vi "Get Movie Paths.vi"(8 "error in (no error)":errorcluster, 11 "Protocol in":refnum<class "Protocol.lvclass">) -> (0 "error out":errorcluster, 2 "Paths":path[](array[path]), 3 "Protocol out":refnum<class "Protocol.lvclass">)   [LabVIEW 2023]
uses:
  Protocol.lvclass
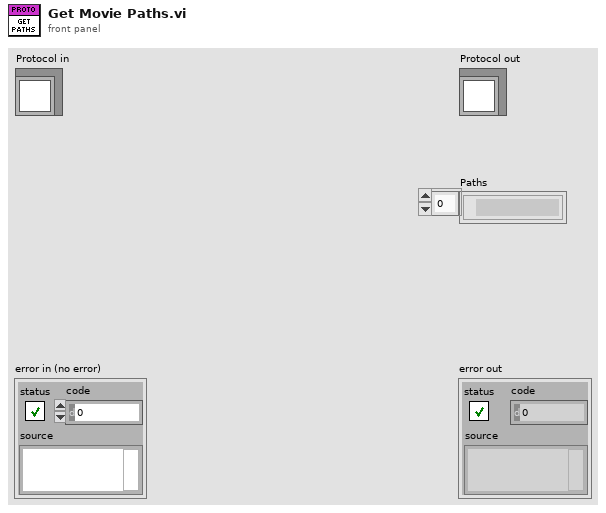
[diagram p1: front panel]
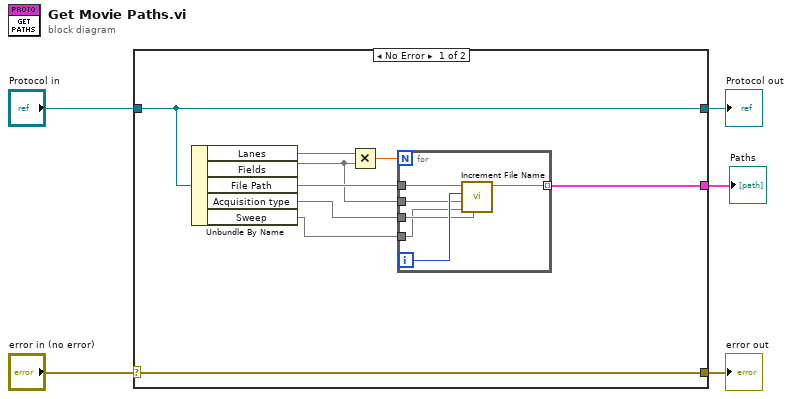
[diagram p0: block diagram]
diagram:
  n1 = case shown="No Error" "error in (no error)" {
    selector: "error in (no error)" -> [w14 w22]
    tunnel: [w14 w22] -> w4
    tunnel: [w13 w21] -> w2
    tunnel: "Protocol in" -> [w13 w21]
    tunnel: [w7 _] -> w1
    frame No Error {
      n2 = Unbundle By Name(w13) -> ("Lanes"=w11, "Fields"=w8, "File Path"=w12, "Acquisition type"=w9, "Sweep"=w6)
      n3 = Multiply(x=w11, y=w8) -> (x*y=w10:dbl)
      n4 = for {
        N: w10 -> [_]
        tunnel: w12 -> [w20]
        tunnel: w8 -> [w18]
        tunnel: w9 -> [w17]
        tunnel: [w16] -> w7 mode=indexing
        tunnel: w6 -> [w15]
        i -> [w19]
        n5 = call "Increment File Name.vi"(6:w17, 8:w15, 9:w18, "Movie Index"=w19, "Movie Series In"=w20) -> (3:w16)  [unwired: 5 in, 1 out]
      }
    }
    frame Error {
    }
  }
  "error out" <- w4
  "Protocol out" <- w2
  "Paths" <- w1
